vi "fpga_Phasor Measurement (M Class_60Hz).vi"(0 "resampled data":T3, 1 "number of channels":T2=1 items=["1"=1, "2"=2, "3"=3, "4"=4, "5"=5, "6"=6, "7"=7, "8"=8, "9"=9, "10"=10, "11"=11, "12"=12, "13"=13, "14"=14, "15"=15, "16"=16], 2 "Memory In":refnum<k21>="coefROM", 5 "reporting rate":i16, 9 "input valid? (T)":bool=TRUE, 12 "ready for output? (T)":bool=TRUE) -> (4 "output data":T1 {"timestamp [s]" format="%#.6g"; "phase [pi]" format="%#.6g"}, 10 "output valid":bool, 14 "ready for input":bool, 15 "error":i32)   [LabVIEW 2013, in "NI_EP_PMU_FPGA.lvlib"]
doc: "Computes the instantaneous magnitude, phase, and frequency values of the fundamental frequency component in an even-angle signal, at an output rate of 24 samples per cycle."
uses:
  <vilib>/addons/Electrical Power/PMU/NI_EP_PMU_FPGA.lvlib
  <vilib>/addons/Electrical Power/PQ/Resampling/FPGA/subVIs/fpga_Resampled.ctl
  <vilib>/addons/Electrical Power/PQ/Resampling/FPGA/subVIs/fpga_NofCH.ctl
  <vilib>/addons/Electrical Power/PMU/FPGA/subVIs/fpga_OutputDataType.ctl
  <vilib>/addons/Electrical Power/PMU/FPGA/subVIs/fpga_Reporting Rate Configuration.ctl
  <vilib>/addons/Electrical Power/PQ/Resampling/NI_EP_Resample_FPGA.lvlib
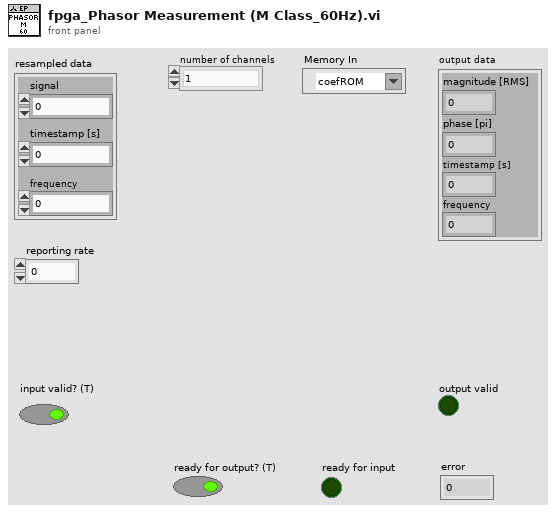
[diagram p1: front panel]
types:
  T1 = typedef "NI_EP_PMU_FPGA.lvlib/fpga_OutputDataType.ctl" = cluster{"magnitude [RMS]":fxp<+,32,6>, "phase [pi]":fxp<+/-,32,2>, "timestamp [s]":fxp<+,64,32>, "frequency":fxp<+,32,8>}
  T2 = typedef "NI_EP_Resample_FPGA.lvlib/fpga_NofCH.ctl" = u8
  T3 = typedef "NI_EP_Resample_FPGA.lvlib/fpga_Resampled.ctl" = cluster{"signal":fxp<+/-,32,3>, "timestamp [s]":fxp<+,64,32>, "frequency":fxp<+,32,8>}
  T4 = typedef "NI_EP_PMU_FPGA.lvlib/fpga_Reporting Rate Configuration.ctl" = enum16{"50Hz:50 reporting rate", "50Hz:25 reporting rate", "50Hz:10 reporting rate", "60Hz:60 reporting rate", "60Hz:30 reporting rate", "60Hz:20 reporting rate", "60Hz:15 reporting rate", "60Hz:12 reporting rate", "60Hz:10 reporting rate"}
  T5 = cluster{"rms magnitude":fxp<+,32,6>, "phase":fxp<+/-,32,2>, "Time Stamp out":fxp<+,64,32>, "Frequency output":fxp<+,32,8>}
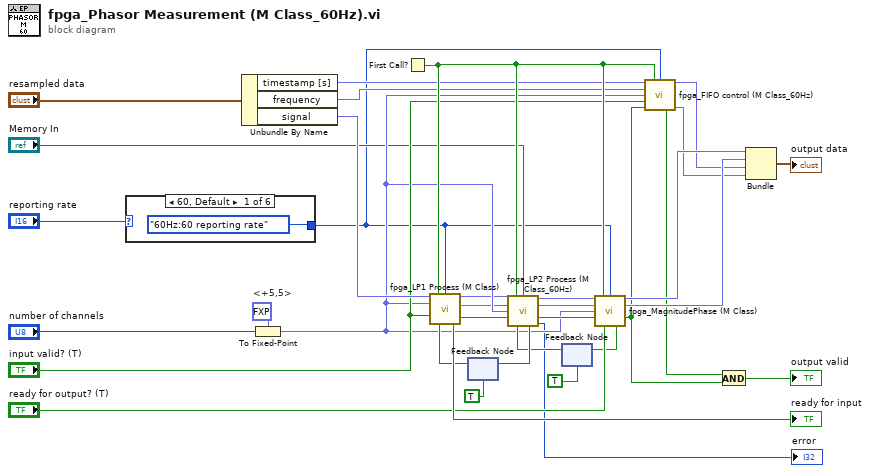
[diagram p0: block diagram]
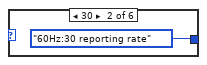
[diagram p2: hidden frame]
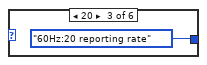
[diagram p3: hidden frame]
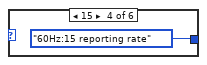
[diagram p4: hidden frame]
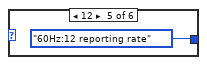
[diagram p5: hidden frame]
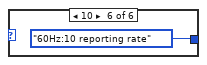
[diagram p6: hidden frame]
diagram:
  w21 = fxp<+,5,5> 0.0  # <+5,5>
  n1 = case shown="60, Default" "reporting rate" {
    tunnel: [fpga_Reporting_Rate_Configuration."60Hz:60 reporting rate" ("filter delay constant") fpga_Reporting_Rate_Configuration."60Hz:30 reporting rate" ("filter delay constant") fpga_Reporting_Rate_Configuration."60Hz:20 reporting rate" ("filter delay constant") fpga_Reporting_Rate_Configuration."60Hz:15 reporting rate" ("filter delay constant") fpga_Reporting_Rate_Configuration."60Hz:12 reporting rate" ("filter delay constant") fpga_Reporting_Rate_Configuration."60Hz:10 reporting rate" ("filter delay constant")] -> w2
    frame 60, Default {
    }
    frame 30 {
    }
    frame 20 {
    }
    frame 15 {
    }
    frame 12 {
    }
    frame 10 {
    }
  }
  n2 = Unbundle By Name("resampled data") -> ("timestamp [s]"=w11:fxp<+,64,32>, "frequency"=w12:fxp<+,32,8>, "signal"=w22:fxp<+/-,32,3>)
  n3 = To Fixed-Point(fixed-point type=w21, number="number of channels") -> (fixed-point=w13:fxp<+,5,5>)
  n4 = First Call?() -> (First Call?: T/F=w18:bool)
  n5 = feedback #1(TRUE ("ready for input")) -> (w29:bool)
  n6 = call <vilib>:"fpga_LP1 Process (M Class).vi"("input data"=w22, "reset"=w18, "filter delay constant"=w2, "Ch"=w13, "input valid"="input valid? (T)", "ready for output"=w29) -> ("re"=w8:fxp<+/-,32,5>, "im"=w7:fxp<+/-,32,5>, "output valid"=w28:bool, "ready for input"=→"ready for input":bool)  [unwired: 6 in]
  n7 = feedback #2(TRUE ("ready for input")) -> (w24:bool)
  n8 = call <vilib>:"fpga_LP2 Process (M Class_60Hz).vi"("re"=w8, "reset"=w18, "Memory In"="Memory In", "im"=w7, "#Ch"=w13, "input valid"=w28, "ready for output"=w24) -> ("re filtered"=w10:fxp<+/-,32,6>, "im filtered"=w9:fxp<+/-,32,6>, "output valid"=w26:bool, "ready for input"=w30:bool, "error"=→"error":i32)  [unwired: 4 in]
  n9 = feedback-in #1(w30) -> ()
  n10 = call <vilib>:"fpga_MagnitudePhase (M Class).vi"("re"=w10, "reset"=w18, "filter delay constant"=w2, "im"=w9, "Ch"=w13, "input valid"=w26, "ready for output"="ready for output? (T)") -> ("rms magnitude"=w20:fxp<+,32,6>, "phase"=w19:fxp<+/-,32,2>, "output valid"=w15:bool, "ready for input"=w25:bool)  [unwired: 5 in]
  n11 = feedback-in #2(w25) -> ()
  n12 = call <vilib>:"fpga_FIFO control (M Class_60Hz).vi"("Time stamp"=w11, "reset"=w18, "filter delay constant"=w2, "Frequency"=w12, "#ch"=w13, "PMU VI input valid"="input valid? (T)", "PMU VI output valid"=w15) -> ("Time Stamp out"=w17:fxp<+,64,32>, "data valid?"=w3:bool, "Frequency output"=w16:fxp<+,32,8>)  [unwired: 6 in]
  n13 = And(x=w3, y=w15) -> (x .and. y?=→"output valid":bool)
  n14 = Bundle("rms magnitude"=w20, "phase"=w19, "Time Stamp out"=w17, "Frequency output"=w16) -> (→"output data":T5)  [unwired: 1 in]
